vi "2Darray2String_UDP.vi"(2 "NumOfCH":i32=8, 3 "NumberOfSamples":i32, 4 "Waveform Graph":dbl[][](graph)) -> (0 "UDP_StringLength":i32, 1 "UDP_String":string)   [LabVIEW 2012]
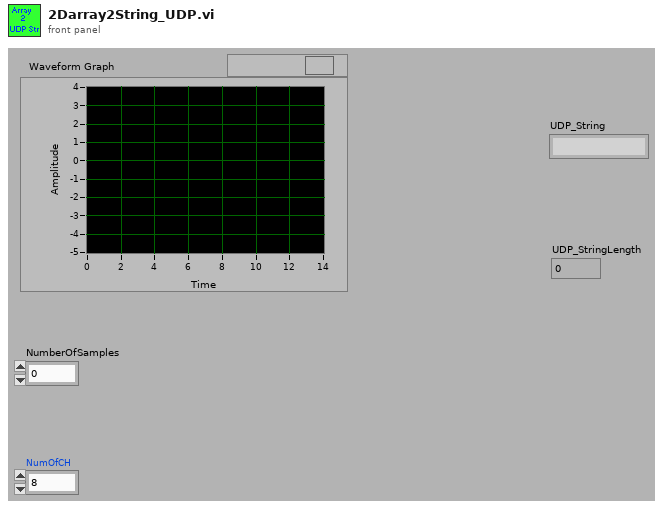
[diagram p1: front panel]
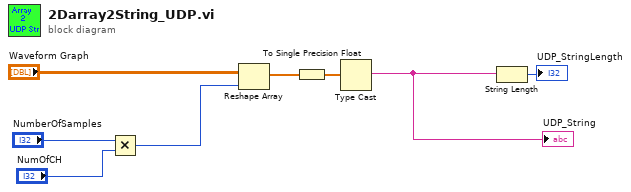
[diagram p0: block diagram]
diagram:
  n1 = Multiply(x="NumberOfSamples", y="NumOfCH") -> (x*y=w2:i32)
  n2 = Reshape Array("Waveform Graph", w2) -> (w1:dbl[])
  n3 = To Single Precision Float(number=w1) -> (single precision float=w6:sgl[])
  n4 = Type Cast(x=w6) -> (*(type *) &x=w8:string)  [unwired: 1 out]
  "UDP_String" <- w8
  n5 = String Length(string=w8) -> (length=→"UDP_StringLength":i32)
